vi "Keep Window Frontmost.vi"(8 "error in (no error)":errorcluster, 10 "Topmost?":bool, 11 "hWnd":i32) -> (0 "error out":errorcluster)   [LabVIEW 2020, in "PicoG-Processor.lvlib"]
uses:
  PicoG-Processor.lvlib
  user32.dll
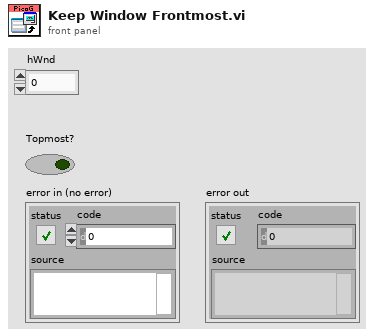
[diagram p1: front panel]
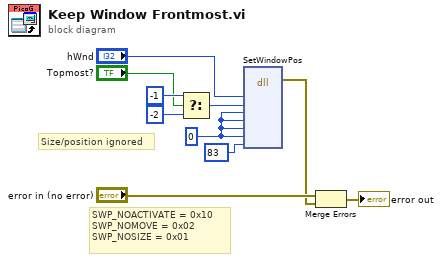
[diagram p0: block diagram]
diagram:
  w2 = 0 ("X")
  # "Size/position ignored"
  # "SWP_NOACTIVATE = 0x10\nSWP_NOMOVE = 0x02\nSWP_NOSIZE = 0x01"
  n1 = Select(t=-1 ("hWndInsertAfter"), s="Topmost?", f=-2 ("hWndInsertAfter")) -> (s? t:f=w5:i32)
  n2 = dll-call lib="user32.dll" fn="SetWindowPos"("hWnd"="hWnd", "hWndInsertAfter"=w5, "X"=w2, "Y"=w2, "cx"=w2, "cy"=w2, "uFlags"=u32 83) -> (error out=w9:errorcluster)  [unwired: 11 in, 1 out]
  n3 = Merge Errors("error in (no error)", w9) -> (→"error out":errorcluster)
